vi "Stop.vi"(8 "error in (no error)":errorcluster, 11 "Encoder Ref In":T1) -> (0 "error out":errorcluster, 3 "Encoder Ref Out":T1)   [LabVIEW 2021, in "Encoder.lvlib"]
doc: "Stops the encoder tick counter. The encoder stops changing the tick counter values."
uses:
  <vilib>/myRIO/Instrument Drivers/Onboard IO/Encoder/Encoder.lvlib
  <vilib>/myRIO/Instrument Drivers/Onboard IO/Encoder/typedefs/Encoder Reference.ctl
  <vilib>/myRIO/Common/Instrument Driver Framework/Utilities/typedefs/myRIO Generic Hardware Reference.ctl
  <vilib>/myRIO/Common/Instrument Driver Framework/Utilities/typedefs/Hardware Version Enum.ctl
  <vilib>/myRIO/Common/Instrument Driver Framework/Utilities/typedefs/myRIO v1.0 Reference.ctl
  <vilib>/myRIO/Common/Instrument Driver Framework/Utilities/typedefs/Generic FPGA Reference.ctl
  <vilib>/myRIO/Common/Instrument Driver Framework/myRIO v1.0/Encoder/typedefs/Encoder Channels Enum.ctl
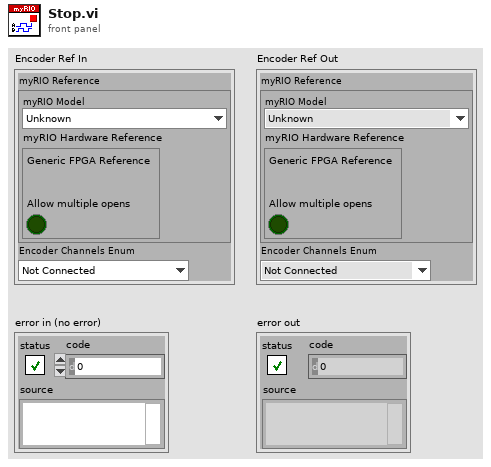
[diagram p1: front panel]
types:
  T1 = typedef "Encoder.lvlib/Encoder Reference.ctl" = cluster{"myRIO Reference":T2, "Encoder Channels Enum":T6}
  T2 = typedef "myRIO Generic Hardware Reference.ctl" = cluster{"myRIO Model":T3, "myRIO Hardware Reference":T4}
  T3 = typedef "Hardware Version Enum.ctl" = enum16{"Unknown", "myRIO-1900", "myRIO-1950", "roboRIO", "NI ELVIS RIO CM", "ELVIS III"}
  T4 = typedef "myRIO v1.0 Reference.ctl" = cluster{"Generic FPGA Reference":T5, "Allow multiple opens":bool}
  T5 = typedef "Generic FPGA Reference.ctl" = refnum<k20>
  T6 = typedef "Encoder Channels Enum.ctl" = enum16{"Not Connected", "C/ENC0", "C/ENC1", "A/ENC", "A/ENC0", "A/ENC1", "A/ENC2", "A/ENC3", "A/ENC4", "A/ENC5", "A/ENC6", "A/ENC7", "A/ENC8", "A/ENC9", "B/ENC", "B/ENC0", "B/ENC1", "B/ENC2", "B/ENC3", "B/ENC4", "B/ENC5", "B/ENC6", "B/ENC7", "B/ENC8", "B/ENC9", "DIO/ENC0", "DIO/ENC1", "DIO/ENC2", "DIO/ENC3", "DIO/ENC4"}
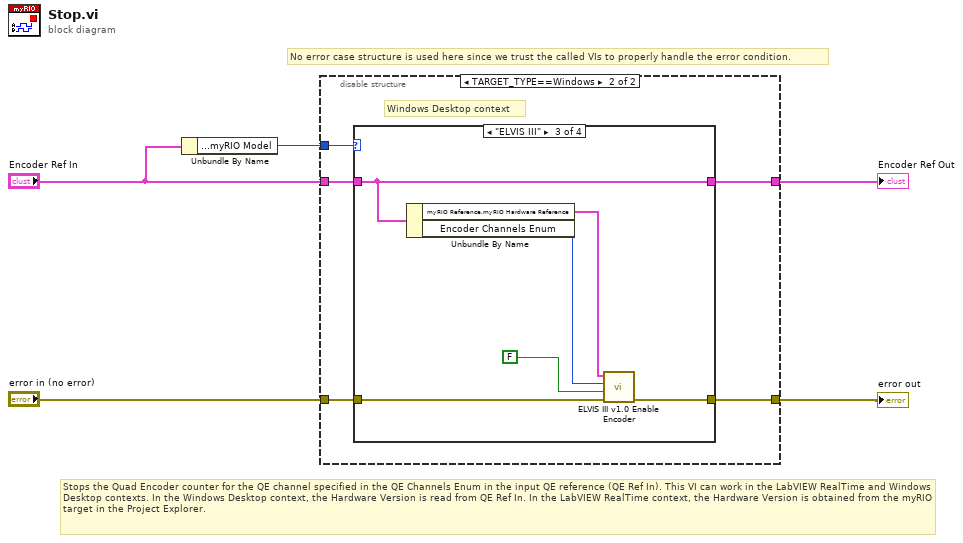
[diagram p0: block diagram]
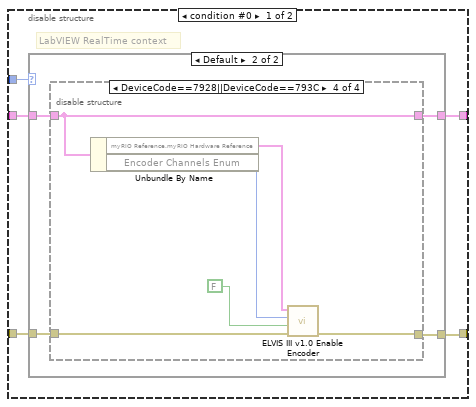
[diagram p2: hidden frame]
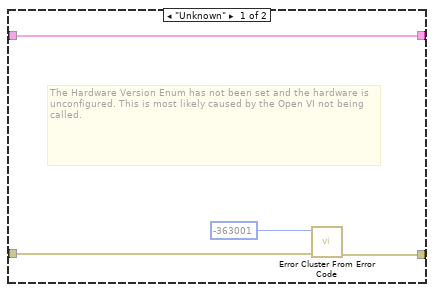
[diagram p3: hidden frame]
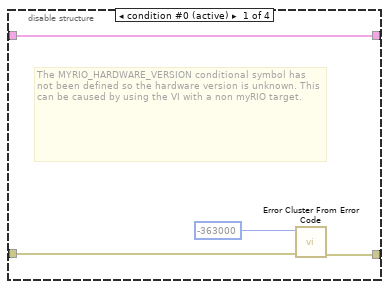
[diagram p4: hidden frame]
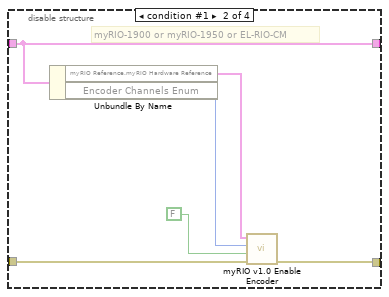
[diagram p5: hidden frame]
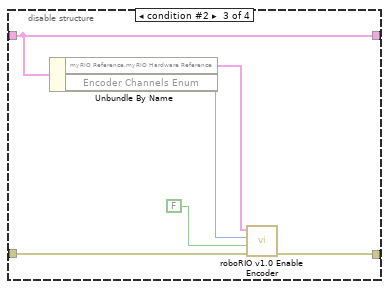
[diagram p6: hidden frame]
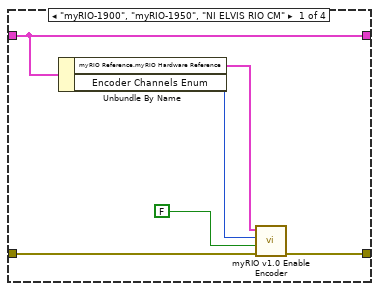
[diagram p7: hidden frame]
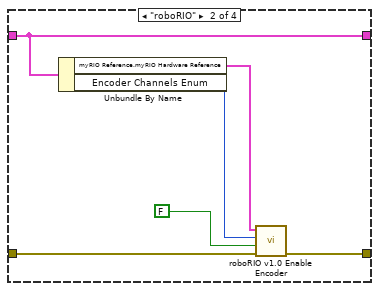
[diagram p8: hidden frame]
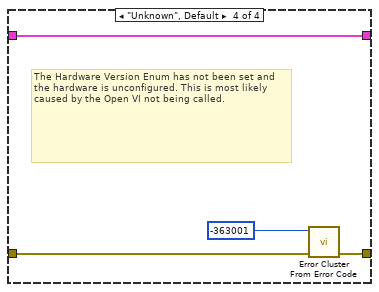
[diagram p9: hidden frame]
diagram:
  # "No error case structure is used here since we trust the called VIs to properly handle the error condition."
  # "Stops the Quad Encoder counter for the QE channel specified in the QE Channels Enum in the input QE reference (QE Ref In). This VI can work in the LabVIEW RealTime and Windows Desktop contexts. In the Windows Desktop context, the Hardware Version is read from QE Ref In. In the LabVIEW RealTime context, the Hardware Version is obtained from the myRIO target in the Project Explorer."
  n1 = Unbundle By Name("Encoder Ref In") -> ("myRIO Reference.myRIO Model"=w1:T3)
  n2 = disable-structure shown="TARGET_TYPE==Windows" {
    disable-tunnel: [w10 w45] -> w2
    disable-tunnel: "Encoder Ref In" -> [w9 w42]
    disable-tunnel: "error in (no error)" -> [w8 w44]
    disable-tunnel: [w7 w43] -> w3
    disable-tunnel: w1 -> [w6 w41]
    frame condition #0 {
      # "LabVIEW RealTime context"
      n3 = case shown="Default" w6 {
        tunnel: [w13 w18] -> w10
        tunnel: w9 -> [w11 w17]
        tunnel: w8 -> [w12 w16]
        tunnel: [w11 w15] -> w7
        frame "Unknown" {
          # "The Hardware Version Enum has not been set and the hardware is unconfigured. This is most likely caused by the Open VI not being called."
          n4 = call <vilib>:"Error Cluster From Error Code.vi"("error in (no error)"=w12, "error code (0)"=-363001) -> ("error out"=w13:errorcluster)  [unwired: 7 in]
        }
        frame Default {
          n5 = disable-structure shown="DeviceCode==7928||DeviceCode==793C" {
            disable-tunnel: w17 -> [w19 w27 w33 w37]
            disable-tunnel: [w22 w25 w31 w36] -> w18
            disable-tunnel: w16 -> [w20 w26 w32 w35]
            disable-tunnel: [w19 w27 w33 w37] -> w15
            frame condition #0 (active) {
              # "The MYRIO_HARDWARE_VERSION conditional symbol has not been defined so the hardware version is unknown. This can be caused by using the VI with a non myRIO target."
              n6 = call <vilib>:"Error Cluster From Error Code.vi"("error in (no error)"=w20, "error code (0)"=-363000) -> ("error out"=w22:errorcluster)  [unwired: 7 in]
            }
            frame condition #1 {
              # "myRIO-1900 or myRIO-1950 or EL-RIO-CM"
              n7 = Unbundle By Name(w27) -> ("myRIO Reference.myRIO Hardware Reference"=w28:T4, "Encoder Channels Enum"=w24:T6)
              n8 = call <vilib>:"myRIO v1.0 Enable Encoder.vi"("error in (no error)"=w26, "Enable"=FALSE, "Channel"=w24, "myRIO Ref In"=w28) -> ("error out"=w25:errorcluster)  [unwired: 6 in, 1 out]
            }
            frame condition #2 {
              n9 = Unbundle By Name(w33) -> ("myRIO Reference.myRIO Hardware Reference"=w34:T4, "Encoder Channels Enum"=w30:T6)
              n10 = call <vilib>:"roboRIO v1.0 Enable Encoder.vi"("error in (no error)"=w32, "Enable"=FALSE, "Channel"=w30, "myRIO Ref In"=w34) -> ("error out"=w31:errorcluster)  [unwired: 6 in, 1 out]
            }
            frame condition #3 {
              n11 = Unbundle By Name(w37) -> ("myRIO Reference.myRIO Hardware Reference"=w40:T4, "Encoder Channels Enum"=w39:T6)
              n12 = call <vilib>:"ELVIS III v1.0 Enable Encoder.vi"("error in (no error)"=w35, "Enable"=FALSE, "Channel"=w39, "myRIO Ref In"=w40) -> ("error out"=w36:errorcluster)  [unwired: 6 in, 1 out]
            }
          }
        }
      }
    }
    frame condition #1 (active) {
      # "Windows Desktop context"
      n13 = case shown="\"ELVIS III\"" w41 {
        tunnel: [w49 w55 w59 w67] -> w45
        tunnel: w42 -> [w50 w56 w60 w64]
        tunnel: w44 -> [w48 w54 w58 w65]
        tunnel: [w50 w56 w60 w64] -> w43
        frame "myRIO-1900", "myRIO-1950", "NI ELVIS RIO CM" {
          n14 = Unbundle By Name(w50) -> ("myRIO Reference.myRIO Hardware Reference"=w51:T4, "Encoder Channels Enum"=w47:T6)
          n15 = call <vilib>:"myRIO v1.0 Enable Encoder.vi"("error in (no error)"=w48, "Enable"=FALSE, "Channel"=w47, "myRIO Ref In"=w51) -> ("error out"=w49:errorcluster)  [unwired: 6 in, 1 out]
        }
        frame "roboRIO" {
          n16 = Unbundle By Name(w56) -> ("myRIO Reference.myRIO Hardware Reference"=w57:T4, "Encoder Channels Enum"=w53:T6)
          n17 = call <vilib>:"roboRIO v1.0 Enable Encoder.vi"("error in (no error)"=w54, "Enable"=FALSE, "Channel"=w53, "myRIO Ref In"=w57) -> ("error out"=w55:errorcluster)  [unwired: 6 in, 1 out]
        }
        frame "ELVIS III" {
          n18 = Unbundle By Name(w60) -> ("myRIO Reference.myRIO Hardware Reference"=w63:T4, "Encoder Channels Enum"=w62:T6)
          n19 = call <vilib>:"ELVIS III v1.0 Enable Encoder.vi"("error in (no error)"=w58, "Enable"=FALSE, "Channel"=w62, "myRIO Ref In"=w63) -> ("error out"=w59:errorcluster)  [unwired: 6 in, 1 out]
        }
        frame "Unknown", Default {
          # "The Hardware Version Enum has not been set and the hardware is unconfigured. This is most likely caused by the Open VI not being called."
          n20 = call <vilib>:"Error Cluster From Error Code.vi"("error in (no error)"=w65, "error code (0)"=-363001) -> ("error out"=w67:errorcluster)  [unwired: 7 in]
        }
      }
    }
  }
  "Encoder Ref Out" <- w3
  "error out" <- w2
